vi "From Data.vi"(0 "Data":refnum<class "Datum.lvclass">[](array[class])) -> (2 "Array":refnum<class "Array.lvclass">)   [LabVIEW 2018, in "Toolkit.lvlib" / "Data.lvlib" / "Array.lvclass"]
uses:
  Array.lvclass
  Datum/Datum.lvclass
  Array.lvclass/Array.ctl
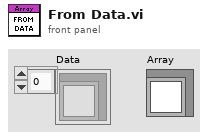
[diagram p1: front panel]
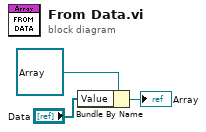
[diagram p0: block diagram]
diagram:
  n1 = Bundle By Name(cluster=refnum<class "Array.lvclass"> refnum ("Toolkit.lvlib:Data.lvlib:Array.lvclass"), "Value"="Data") -> (→"Array":refnum<class "Array.lvclass">)
